vi "Display control.vi"(7 "Cursor Blink":bool, 8 "error in (no error)":errorcluster, 9 "Enable Display":bool, 10 "Enable Cursor":bool, 11 "Refnum in":T1) -> (0 "error out":errorcluster, 3 "Refnum out":T1)   [LabVIEW 2019, in "HD44780.lvlib"]
uses:
  HD44780.lvlib
  FPGA VI Reference.ctl
  <vilib>/Utility/error.llb/Error Cluster From Error Code.vi
  <vilib>/rvi/errors/niLvFpgaAdjustHostInterfaceError.vi
  <vilib>/rvi/interface/nirviReadWriteControl/nirviReadWriteControl.xnode
  NiFpgaLv.dll
  <vilib>/rvi/interface/Simulation/niFpgaSimulationCallBeginRW.vi
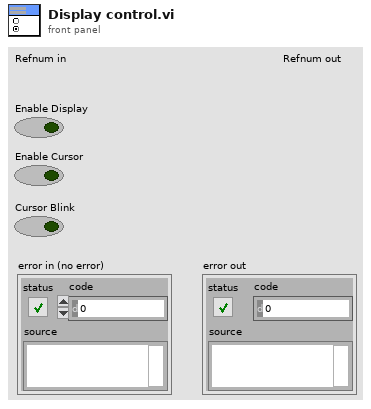
[diagram p1: front panel]
types:
  T1 = typedef "FPGA VI Reference.ctl" = refnum<k20>
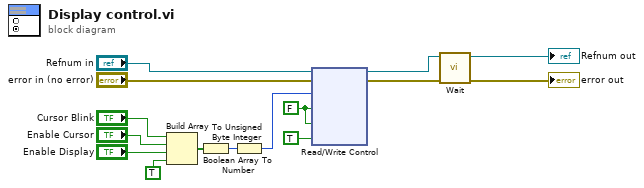
[diagram p0: block diagram]
diagram:
  w14 = FALSE ("RS")
  n1 = Build Array("Cursor Blink", "Enable Cursor", "Enable Display", TRUE ("element")) -> (w11:bool[])
  n2 = Boolean Array To Number(Boolean array=w11) -> (number=w12:u32)
  n3 = To Unsigned Byte Integer(number=w12) -> (unsigned 8bit integer=w13:u8)
  n4 = xnode "Read/Write Control"("FPGA VI Reference In"="Refnum in", "error in"="error in (no error)", "Data In"=w13, "RS"=w14, "R/W"=w14, "Enable"=TRUE) -> ("FPGA VI Reference Out"=w2:T1, "error out"=w4:errorcluster)
  n5 = call "Wait.vi"("error in (no error)"=w4, "Refnum in"=w2) -> ("error out"=→"error out":errorcluster, "Refnum out"=→"Refnum out":T1)  [unwired: 8 in]
